vi "Synchronize Control Panel.vi"(8 "error in (no error)":errorcluster, 11 "LakeShore 340 in":refnum<class "LakeShore 340.lvclass">) -> (0 "error out":errorcluster, 3 "LakeShore 340 out":refnum<class "LakeShore 340.lvclass">)   [LabVIEW 2015, in "LakeShore 340.lvclass"]
uses:
  LakeShore 340.lvclass
  LakeShore340 Front Panel Data.ctl
  LakeShore340 Heater Ranges.ctl
  Neocera/Neocera Set Point Aproach.ctl
  Instrument/Read VISA Resource.vi
  Instrument/Write VISA Resource.vi
  OO Devices/Device/Device.lvclass
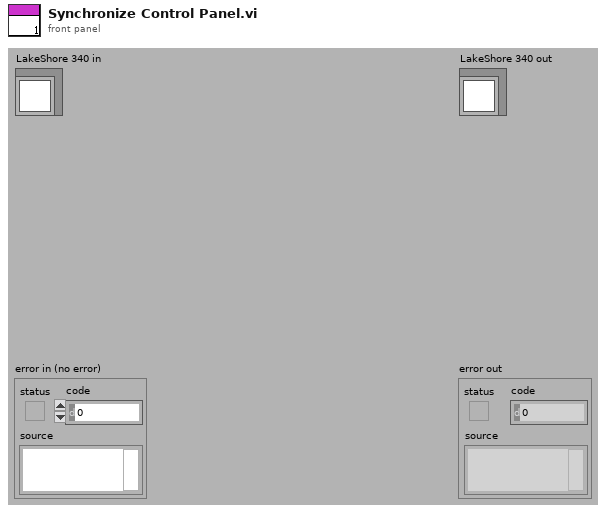
[diagram p1: front panel]
types:
  T1 = typedef "LakeShore340 Front Panel Data.ctl" = cluster{"Record heater":bool, "A":bool, "B":bool, "Record RAW":bool, "Set point":dbl, "Set Heater Range":T2, "Approach":T3, "Ramp rate, K/min":dbl, "C":bool, "D":bool}
  T2 = typedef "LakeShore340 Heater Ranges.ctl" = enum16{"0 (Off)", "1 (5 mW)", "2 (50 mW)", "3 (500 mW)", "4 (5 W)", "5 (50 W)"}
  T3 = typedef "Neocera Set Point Aproach.ctl" = enum16{"Instant", "Ramp"}
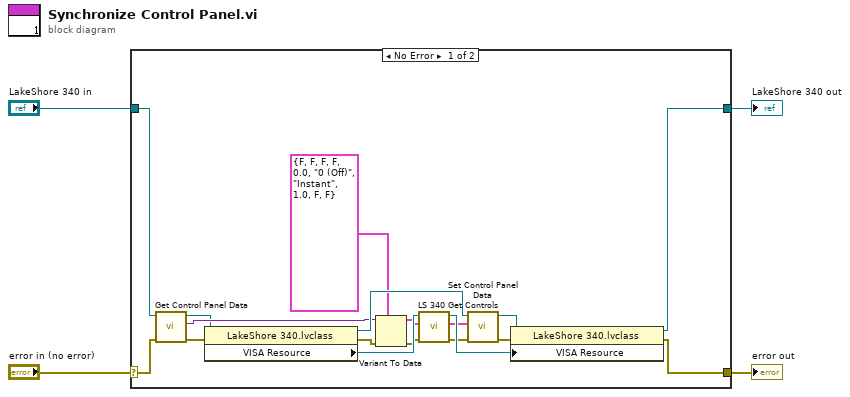
[diagram p0: block diagram]
diagram:
  n1 = case shown="No Error" "error in (no error)" {
    selector: "error in (no error)" -> [w8 w24]
    tunnel: [w7 w24] -> w3
    tunnel: [w5 w23] -> w1
    tunnel: "LakeShore 340 in" -> [w6 w23]
    frame No Error {
      n2 = call-dynamic "Get Control Panel Data.vi"("error in (no error)"=w8, "Device in"=w6) -> ("error out"=w16:errorcluster, "Data"=w13:variant, "Device out"=w9:refnum<class "LakeShore 340.lvclass">)  [unwired: 7 in]
      n3 = property class="LakeShore 340.lvclass"(reference=w9, error in=w16) -> (reference out=w18:refnum<class "LakeShore 340.lvclass">, error out=w17:errorcluster, "VISA Resource"=w22:refnum<visa-resource-name>)
      n4 = Variant To Data(error in=w17, type=T1 {"Record heater"=FALSE, "A"=FALSE, "B"=FALSE, "Record RAW"=FALSE, "Set point"=0.0, "Set Heater Range"=enum."0 (Off)", "Approach"=enum."Instant", "Ramp rate, K/min"=1.0, "C"=FALSE, "D"=FALSE} ("Data"), Variant=w13) -> (data=w12:T1, error out=w11:errorcluster)
      n5 = call "LS 340 Get Controls.vi"("error in (no error)"=w11, "Control Panel Data"=w12, "VISA resource name"=w22) -> ("error out"=w14:errorcluster, "Control Panel Data Out"=w15:T1, "VISA Resource Name Out"=w21:refnum<visa-resource-name>)  [unwired: 6 in]
      n6 = call "Set Control Panel Data.vi"("error in (no error)"=w14, "Data"=w15, "Device in"=w18) -> ("error out"=w20:errorcluster, "Device out"=w19:refnum<class "LakeShore 340.lvclass">)  [unwired: 7 in]
      n7 = property class="LakeShore 340.lvclass"(reference=w19, error in=w20, "VISA Resource"=w21) -> (reference out=w5:refnum<class "LakeShore 340.lvclass">, error out=w7:errorcluster)
    }
    frame Error {
    }
  }
  "error out" <- w3
  "LakeShore 340 out" <- w1
